vi "LogMsg.vi"(8 "External listbox\nto add items to":refnum<vi>, 9 "Set external listbox":bool, 11 "msg":string) -> ()   [LabVIEW 2011]
uses:
  kernel32.dll
panel:
  in  "Listbox":i32(listbox)
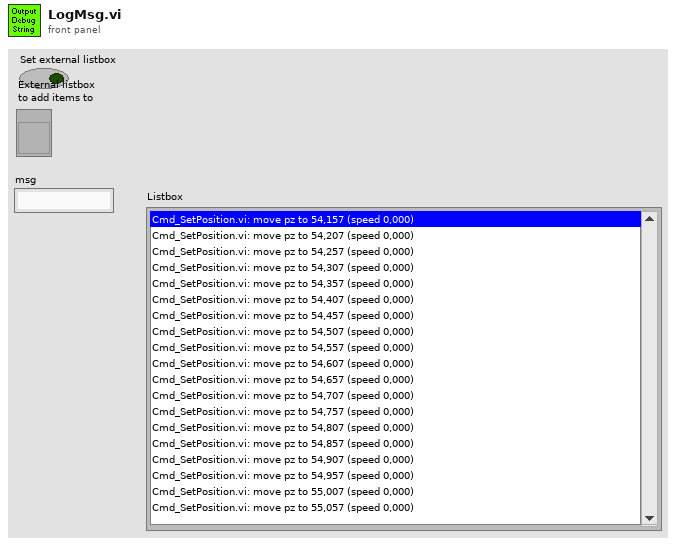
[diagram p1: front panel]
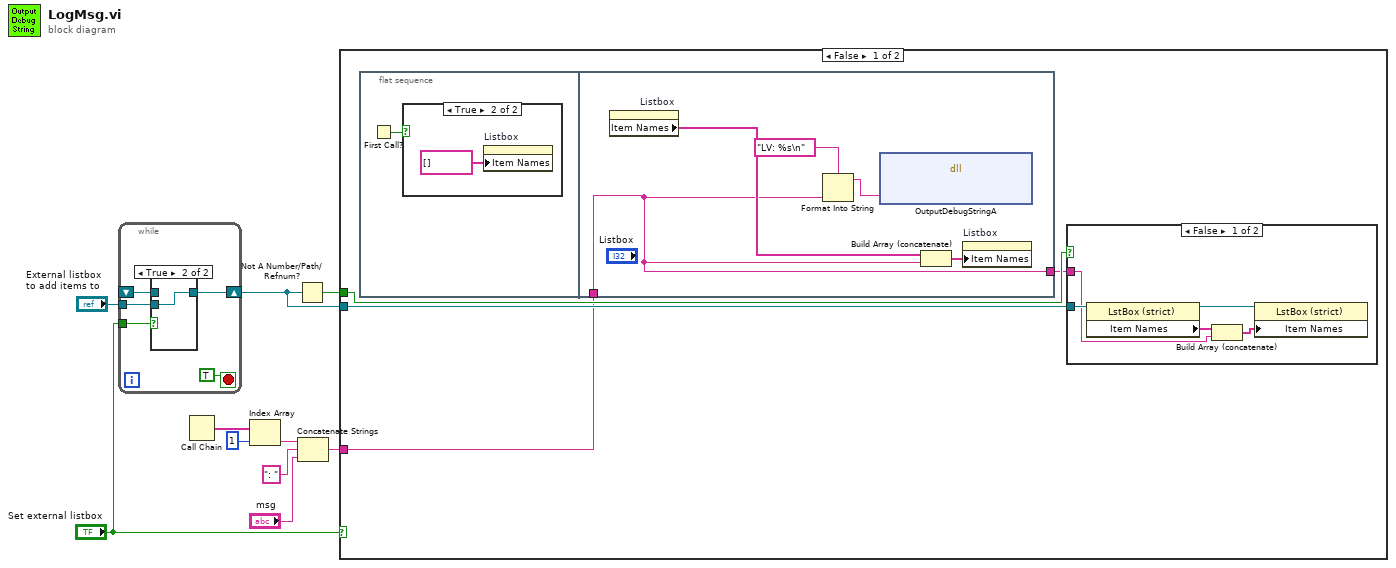
[diagram p0: block diagram]
diagram:
  n1 = while {
    shift-right: [w15] -> w9
    shift-left: _ -> [w13]
    tunnel: "External listbox\nto add items to" -> [w14]
    tunnel: "Set external listbox" -> [w11]
    stop <- TRUE stop-if-true
    n2 = case shown="True" w11 {
      tunnel: [w16 w17] -> w15
      tunnel: w14 -> [_ w17]
      tunnel: w13 -> [w16 _]
      frame False {
      }
      frame True {
      }
    }
  }
  n3 = Call Chain() -> (call chain=w6:string[])
  n4 = Index Array(array=w6, index=1) -> (element=w4:string)
  n5 = Not A Number/Path/Refnum?(number/path/refnum=w9) -> (NaN/Path/Refnum?=w10:bool)
  n6 = Concatenate Strings(w4, ": " ("string"), "msg") -> (w1:string)
  n7 = case shown="False" "Set external listbox" {
    tunnel: w10 -> [w21 _]
    tunnel: w9 -> [w20 _]
    tunnel: w1 -> [w18 _]
    frame False {
      n8 = flat-sequence {
        tunnel: [w30] -> w19
        tunnel: w18 -> [w30]
        frame #0 {
          n9 = First Call?() -> (First Call?: T/F=w27:bool)
          n10 = case shown="True" w27 {
            frame False {
            }
            frame True {
              n11 = property on="Listbox" class="LstBox (strict)"("Item Names"=string[] []) -> ()  [unwired: 2 in, 2 out]
            }
          }
        }
        frame #1 {
          n12 = property on="Listbox" class="LstBox (strict)"() -> ("Item Names"=w32:string[])  [unwired: 2 in, 2 out]
          n13 = Format Into String(format string="LV: %s\n", w30) -> (resulting string=w29:string)  [unwired: 2 in, 1 out]
          n14 = dll-call lib="kernel32.dll" fn="OutputDebugStringA"("msg"=w29) -> ()  [unwired: 5 in, 2 out]
          n15 = Build Array (concatenate)(w32, w30) -> (w33:string[])
          n16 = property on="Listbox" class="LstBox (strict)"("Item Names"=w33) -> ()  [unwired: 2 in, 2 out]
        }
      }
      n17 = case shown="False" w21 {
        tunnel: w20 -> [w26 _]
        tunnel: w19 -> [w24 _]
        frame False {
          n18 = property on="Property Node" class="LstBox (strict)"(reference=w26) -> (reference out=w23:refnum<vi>, "Item Names"=w25:string[])  [unwired: 1 in, 1 out]
          n19 = Build Array (concatenate)(w25, w24) -> (w22:string[])
          n20 = property on="Property Node" class="LstBox (strict)"(reference=w23, "Item Names"=w22) -> ()  [unwired: 1 in, 2 out]
        }
        frame True {
        }
      }
    }
    frame True {
    }
  }
